vi "_Close_Port.vi"(8 "error in (no error)":errorcluster, 11 "Postgres Connector.lvclass":refnum<class "Postgres Connector.lvclass">) -> (0 "error out":errorcluster, 3 "output cluster":refnum<class "Postgres Connector.lvclass">)   [LabVIEW 2020, in "Postgres Connector.lvclass"]
doc: "VI used to close the TCP connection with the server."
uses:
  Postgres Connector.lvclass
  Postgres Connector.lvclass/Postgres Connector.ctl
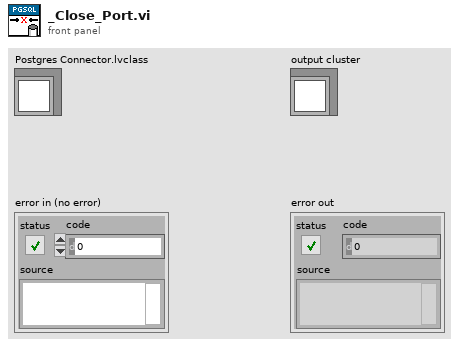
[diagram p1: front panel]
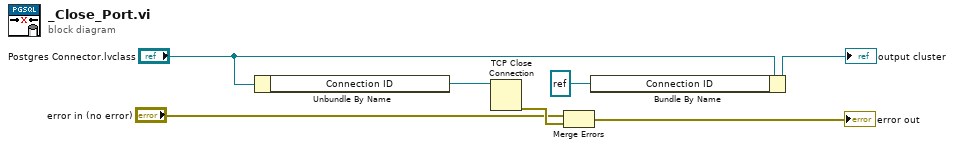
[diagram p0: block diagram]
diagram:
  n1 = Unbundle By Name("Postgres Connector.lvclass") -> ("Connection ID"=w5:refnum<k5>)
  n2 = TCP Close Connection(connection ID=w5) -> (error out=w3:errorcluster)  [unwired: 2 in, 1 out]
  n3 = Merge Errors("error in (no error)", w3) -> (→"error out":errorcluster)
  n4 = Bundle By Name(cluster="Postgres Connector.lvclass", "Connection ID"=refnum<k5> refnum ("connection ID out")) -> (→"output cluster":refnum<class "Postgres Connector.lvclass">)
